vi "断电保存全局.vi"() -> ()   [LabVIEW 2016, in "质控单元.lvlib"]
uses:
  <vilib>/Plasmionique/MB Master/MB_Master/MB_Master.lvclass
panel:
  in  "定时控制":T1
  in  "MB session in":refnum<class "MB_Master.lvclass">
  in  "总氮模块选择":bool=TRUE
  in  "PORT":string="502"
  in  "IP":string="192.168.1.207"
  in  "MB通信方式选择":enum16{"串口", "TCP"}(ring)=enum."TCP"
  in  "Serial Config":T2={"baud rate (bps)"=115200, "stop bits"=10, "parity"=0, "flow control"=0, "timeout"=500, "retries"=1} {"stop bits" items=["1.0"=10, "1.5"=15, "2.0"=20]; "parity" items=["None", "Odd", "Even", "Mark", "Space"]; "flow control" items=["None", "XON/XOFF", "RTS/CTS", "XON/XOFF & RTS/CTS", "DTR/DSR", "XON/XOFF & DTR/DSR"]}
  in  "VISA Resource":refnum<visa-resource-name>="COM8"
  in  "CODCr选择":bool
  in  "CODMn选择":bool=TRUE
  in  "总磷模块选择":bool=TRUE
  in  "氨氮模块":bool=TRUE
  in  "CODCr量程选择":enum32{"H", "L", "AUTO"}(ring)=enum."L"
  in  "CODMn量程选择":enum32{"H", "L", "AUTO"}(ring)=enum."L"
  in  "总磷量程选择":enum32{"H", "L", "AUTO"}(ring)=enum."L"
  in  "总氮量程选择":enum32{"H", "L", "AUTO"}(ring)=enum."L"
  in  "氨氮量程选择":enum32{"H", "L", "AUTO"}(ring)=enum."L"
  # "MBTCP参数"
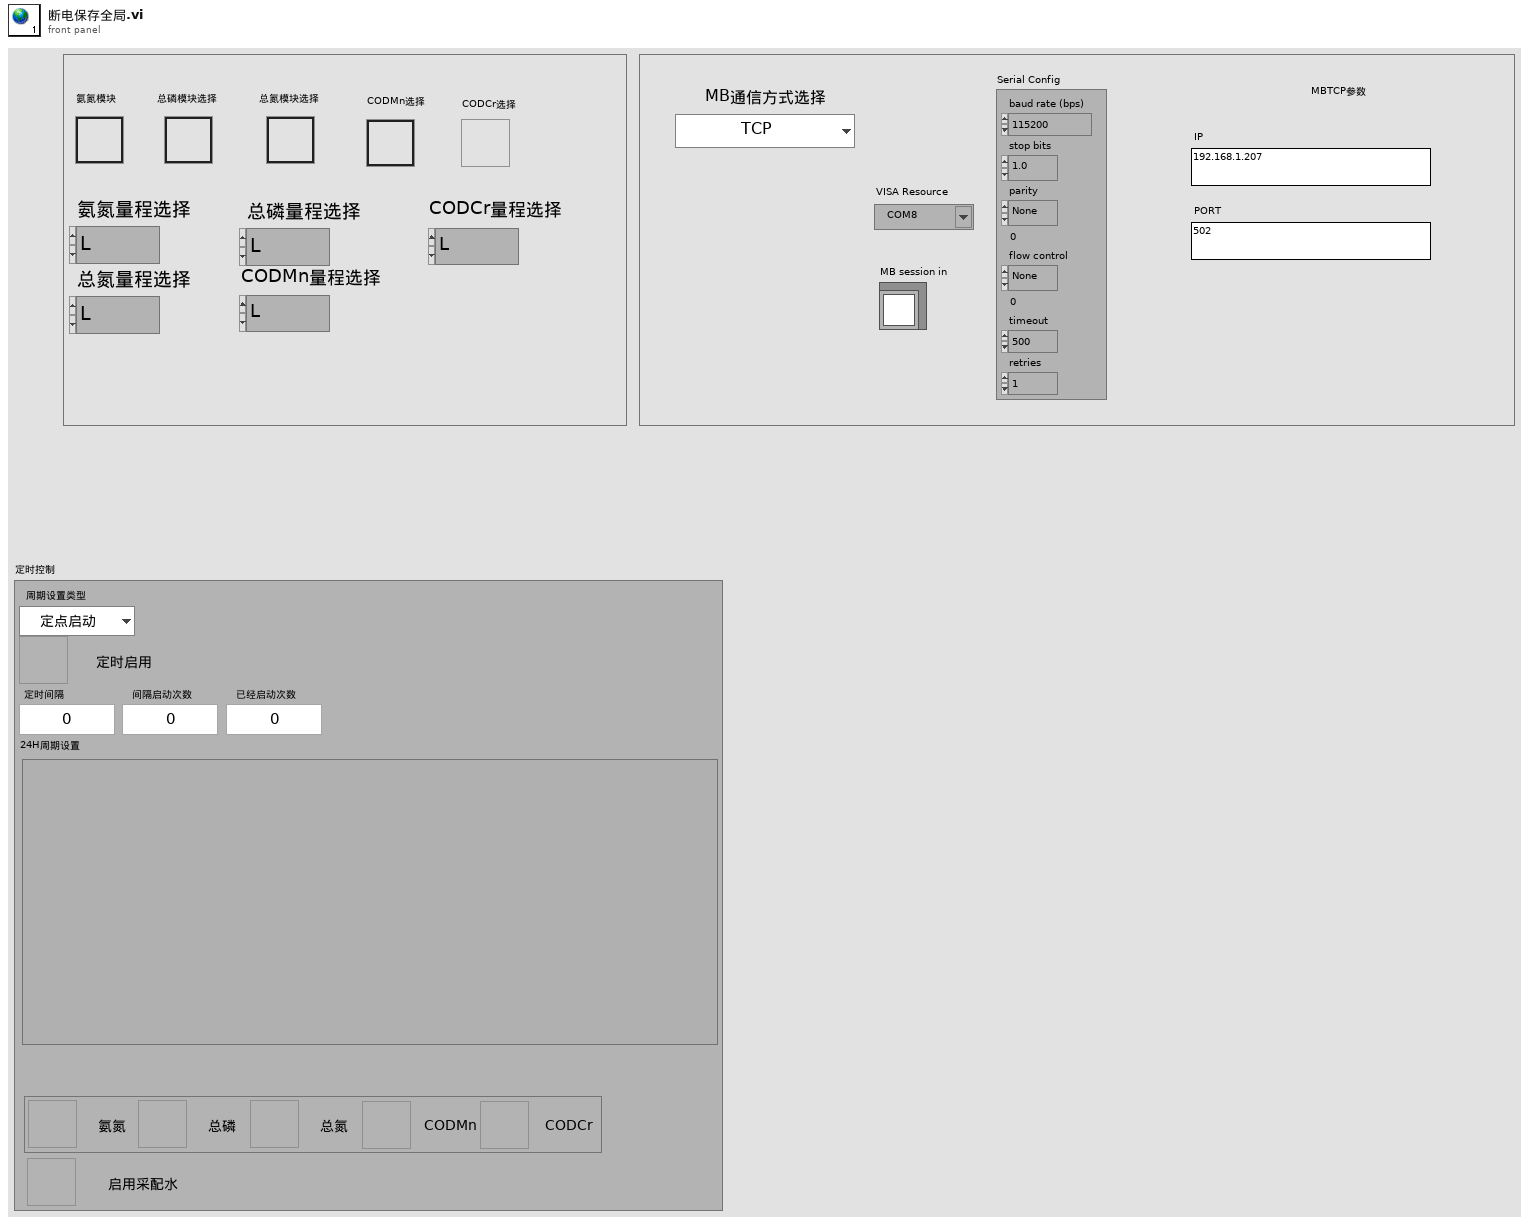
[diagram p1: front panel]
types:
  T1 = cluster{"周期设置类型":enum16{"定点启动", "间隔启动"}, "定时功能启用":bool, "定时间隔":dbl, "间隔启动次数 ":dbl, "已经启动次数 ":dbl, "24H周期设置":bool[], "模块选择":cluster{"氨氮":bool, "总磷":bool, "总氮":bool, "CODMn":bool, "CODCr":bool}, "采配水启用":bool}
  T2 = cluster{"baud rate (bps)":u32, "stop bits":u16, "parity":u16, "flow control":u16, "timeout":u32, "retries":i32}
diagram:
